vi "Main FPGA 5-axis with Limits.vi"() -> ()   [LabVIEW 2013]
uses:
  <vilib>/Motion/MotorControl/_s/nism.interpretControlRegister.stateTransition.ctl
  <vilib>/Platform/TimedLoop/XDataNode/timing_clust.ctl
  <vilib>/Platform/TimedLoop/XDataNode/nitl_modes.ctl
  <vilib>/Platform/TimedLoop/XDataNode/wakeup.ctl
  <vilib>/Motion/MotorControl/_s/nism.digitalInputs.portA.ctl
  <vilib>/rvi/Emulation/niFpgaSctlEmulationGetInTimedLoop.vi
  <vilib>/rvi/Emulation/niFpgaEmulationReportErrorSimple.vi
  <vilib>/rvi/Emulation/niFpgaGetClockAttributes.vi
  <vilib>/rvi/Emulation/niFpgaCriticalErrorInLSC.vi
  Global FPGA.vi
  <vilib>/rvi/eio/common/nirviEmuTemplateMethod_errors.vi
  <vilib>/Motion/SoftMotion/Synchronization/nism.rioScan.generateSyncScan.vi
  <vilib>/rvi/Emulation/niFpgaProcessEmulError.vi
  <vilib>/Motion/MotorControl/_s/nism.interpretControlRegister.indexed.vi
  <vilib>/Motion/MotorControl/_s/nism.generateStatusRegister.indexed.vi
  <vilib>/Motion/MotorControl/_s/nism.mdo.read.positionLoopSyncData.vi
  <vilib>/Motion/MotorControl/_s/nism.mdo.read.splineData.vi
  <vilib>/Motion/MotorControl/_s/nism.splineInterpolation.fxp.3.index.vi
  <vilib>/Motion/MotorControl/_s/nism.mdo.handler.indexed.vi
  <vilib>/Motion/MotorControl/_s/nism.digitalFilter.u8.vi
  <vilib>/Motion/MotorControl/_s/nism.interpretDIOControl.portA.single.2.vi
  <vilib>/Motion/MotorControl/_s/nism.generateDIOStatus.portA.single.vi
  <vilib>/Platform/TimedLoop/XDataNode/XDataNode.xnode
  <vilib>/eio/EIONode/EIONode.xnode
  <vilib>/Motion/MotorControl/NI_SoftMotion_MotorControlIP.lvlib
  <vilib>/Platform/TimedLoop/XDataNode/XDNodeRunTimeDep.lvlib
  <vilib>/Motion/SoftMotion/Synchronization/NI_SoftMotion_Synchronization.lvlib
panel:
  in  "Axis Digital Inputs (U8)":u8[](array[numeric])=[0, 0, 0, 0, 0, 0, 0, 0]
  out "Axis Positions":fxp<+/-,64,32>[](array[numeric])
  in  "STEP or CW? (T=STEP)":bool
  out "Drive Enable":bool[](array[boolean])
  in  "Enable Watchdog":bool
  in  "Pet Watchdog":bool
  in  "Watchdog Timeout Period (ticks)":u64=40000000 format="%.0p"
  out "Watchdog Timed Out?":bool
  out "Time Since Last Pet":u64
  in  "Enable value":bool
  in  "Drive Enable override?":bool
  out "State":T1=enum."Start --> Initializing" caption="state transition"
  in  "Sync Value":bool
  in  "Sync Enable override?":bool
  in  "Invert direction?":bool
  out "Sync is Fault":bool
  out "Sync is Locked":bool
  in  "minimum pulse":u16=40
  # "Synchronization Loop"
  # "Control Status Loop"
  # "Notes: \n1. This VI provides the communication interface between the NI SoftMotion Engine and the LabVIEW FPGA Module. You must compile this VI for a specific FPGA target before use. After compiling, run the VI before running any of the Express VI examples. For information on moving this example to another FPGA target, refer to ni.com/info and enter info code fpgaex.\n\n2. Only use the Reset Axis button if you are unable to communicate with the axis by any other means. This button resets the device state machine and other VIs to a known state. After resetting the axis, switch the NI Scan Engine from Active Mode to Configuration Mode, then back to Active Mode, before attempting to enable the axis."
  # "(These two buttons \nare for testing\npurposes.)"
  # "(These two buttons \nare for testing\npurposes.)"
  # "Step/Direction Loop"
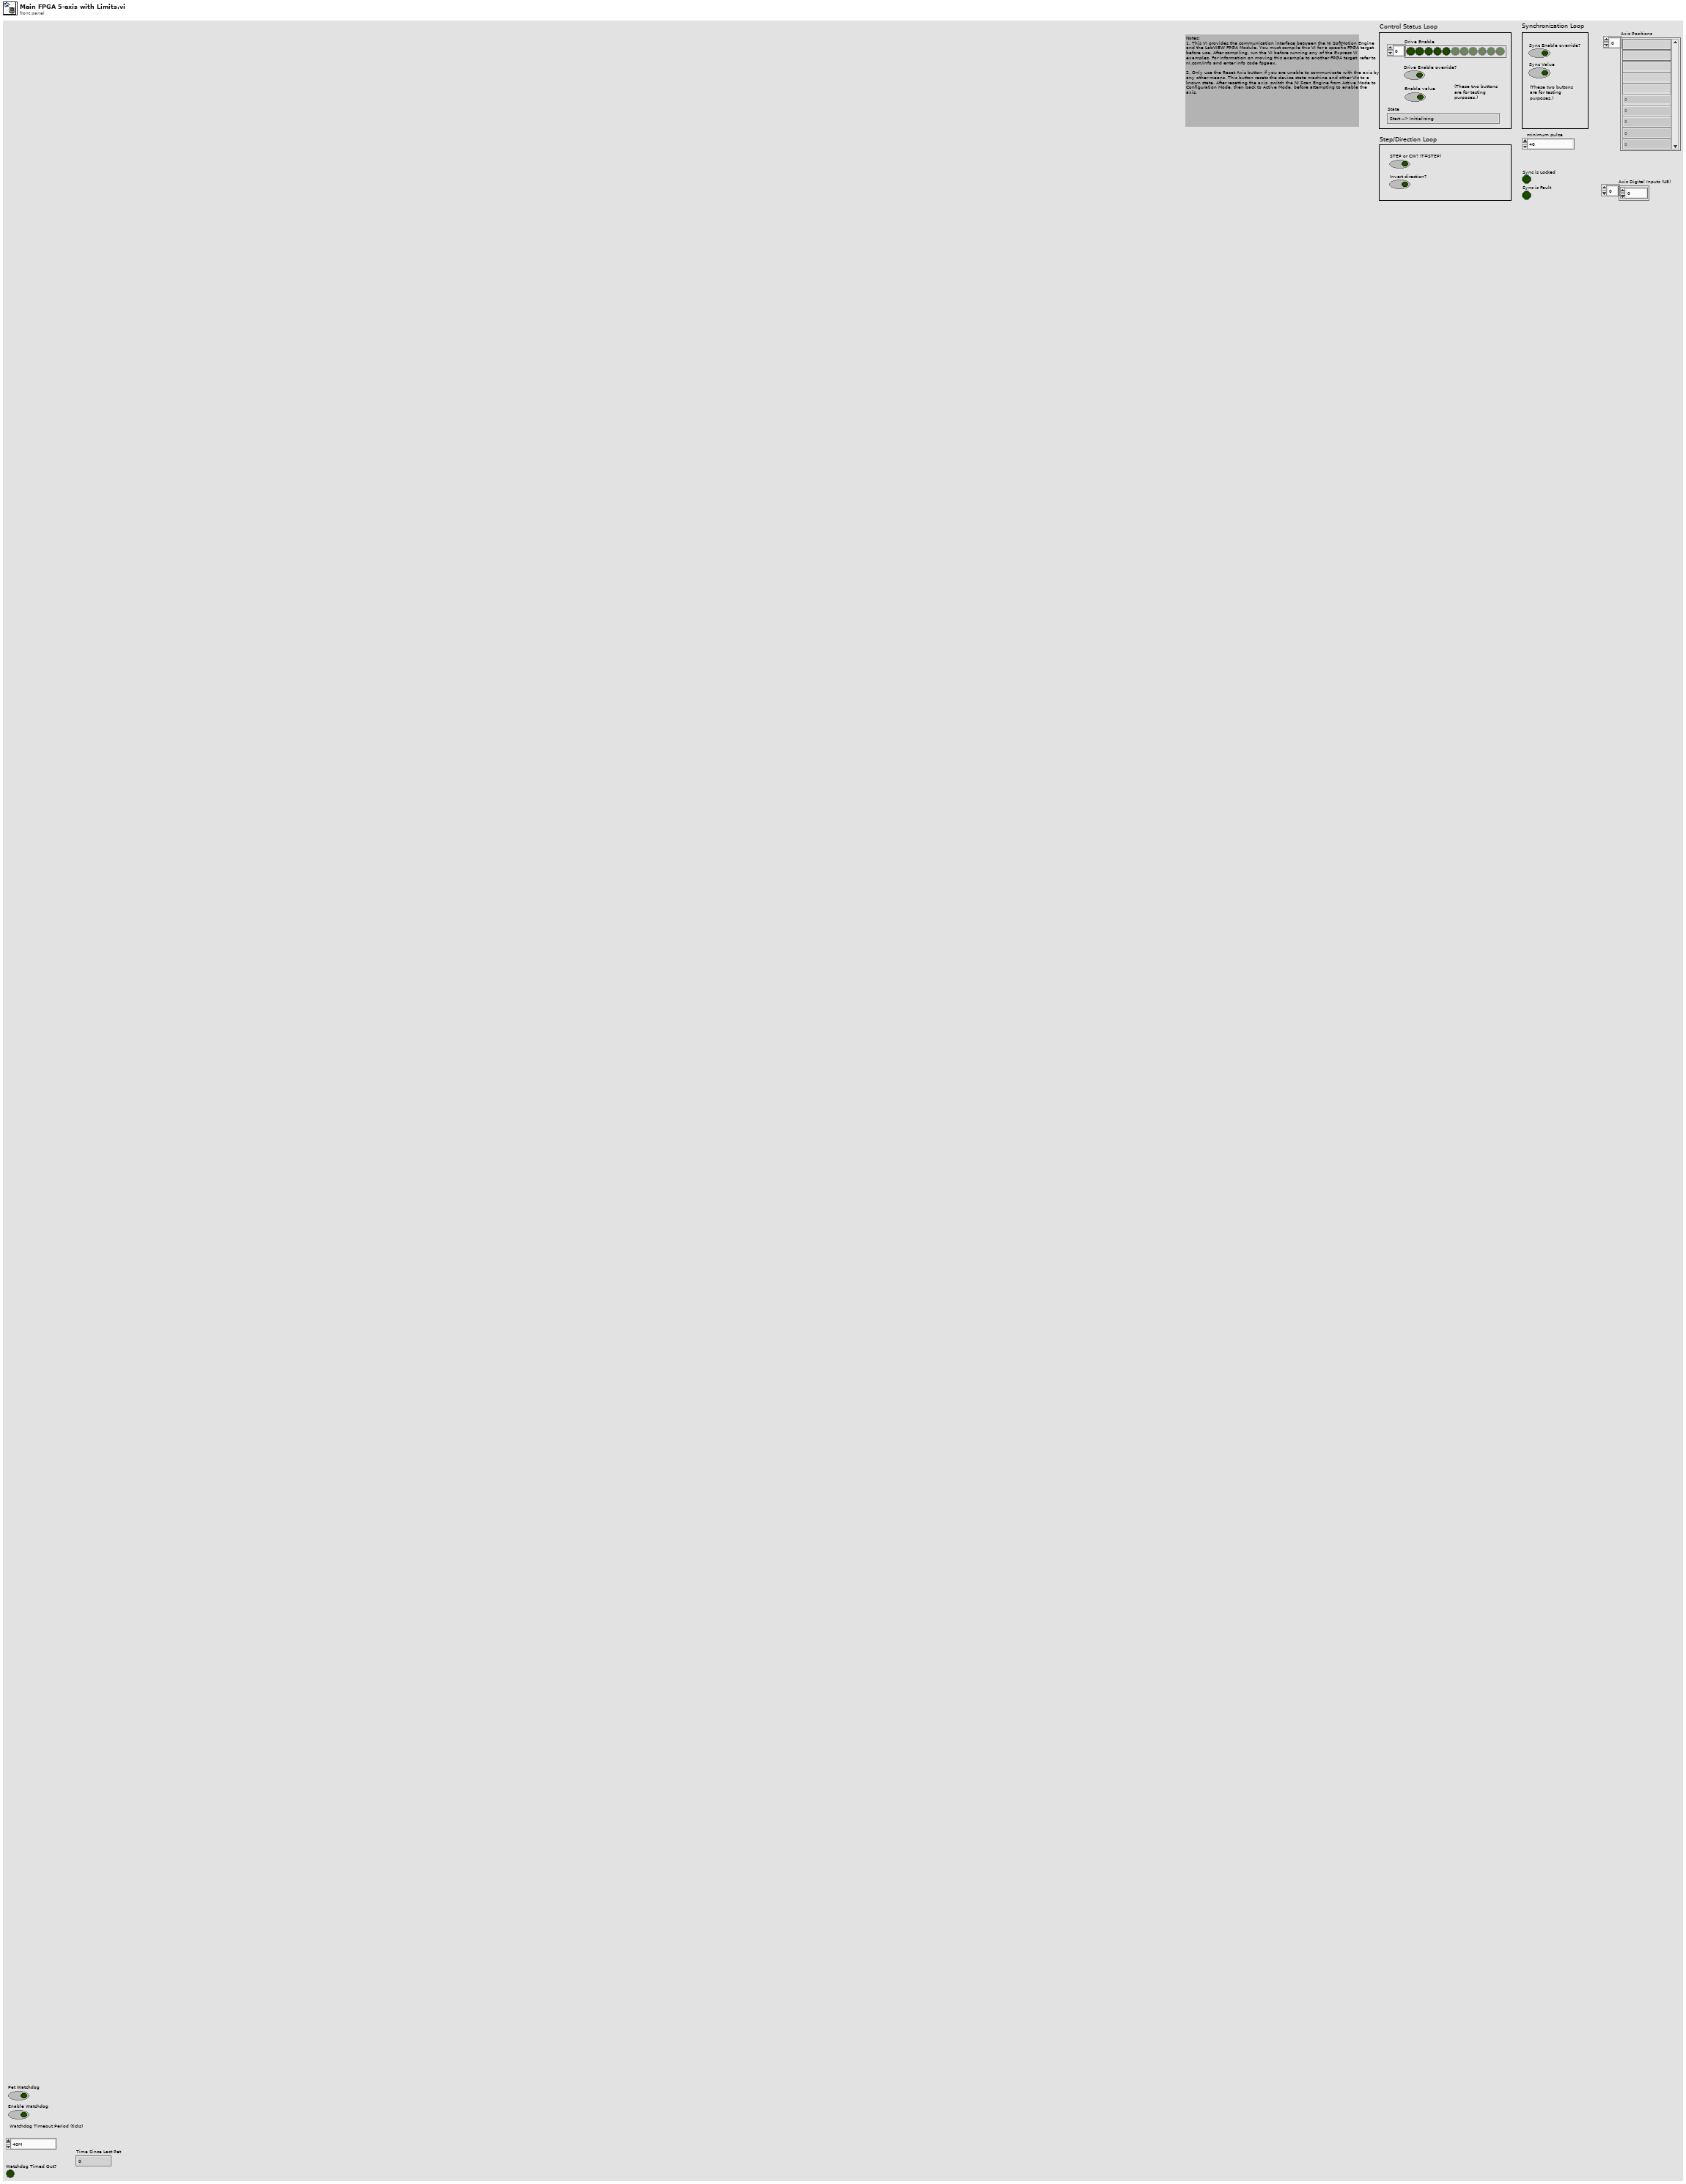
[diagram p1: front panel]
types:
  T1 = typedef "NI_SoftMotion_MotorControlIP.lvlib/nism.interpretControlRegister.stateTransition.ctl" = enum8{"Invalid", "Start --> Initializing", "Initializing --> Disabled", "Disabled --> Ready To Switch On", "Ready To Switch On --> Switched On", "Ready To Switch On --> Disable", "Switched On --> Operation Enable", "Switched On --> Ready To Switch On", "Switched On --> Disabled", "Operation Enable --> Switched On", "Operation Enable --> Ready To Switch On", "Operation Enable --> Disabled", "Fault --> Disabled", "Any --> Fault", "None"}
  T2 = typedef "NI_SoftMotion_MotorControlIP.lvlib/nism.mdo.splineData.ctl" = cluster{"spline type":T3, "traj per/spline per":u16, "spline per/traj per":fxp<+,32,0>}
  T3 = typedef "nism.splineInterpolation.type.ctl" = u16
  T4 = typedef "NI_SoftMotion_Synchronization.lvlib/nism.softmotionScan.timerConfig.ctl" = cluster{"Target Period (clocks)":u16, "Host Period / Target Period":u16}
  T5 = typedef "NI_SoftMotion_Synchronization.lvlib/nism.softmotionScan.timerControl.ctl" = cluster{"SM Scan":bool, "SM Scan Count":u32, "SM Scan Enabled":bool}
  T6 = typedef "XDNodeRunTimeDep.lvlib/timing_clust.ctl" = cluster{"Expected End [f-1]":u64, "Actual End [f-1]":u64, "Finished Late? [f-1]":bool, "Expected End [i-1]":u64, "Actual End [i-1]":u64, "Finished Late? [i-1]":bool, "Expected Start [i]":u64, "Actual Start [i]":u64, "Expected Start [f]":u64, "Actual Start [f]":u64, "Source Name":string, "Structure Name":string, "Period":i64, "Deadline":i64, "Offset":i64, "Start":i64, "Priority":i32, "Timeout":i32, "Mode":T7, "Wakeup Reason":T8, "Error":errorcluster, "Source Type":string, "Secondary Source Type":string, "Global End Time":u64, "Global Start Time":u64, "Frame Duration":u64, "Iteration Duration":u64, "Assigned CPU":i32, "I/O Scan Engine Mode":u32}
  T7 = typedef "XDNodeRunTimeDep.lvlib/nitl_modes.ctl" = enum32{"No Change", "Process missed periods, maintain original phase", "Discard missed periods, maintain original phase", "Process missed periods, ignore original phase", "Discard missed periods, ignore original phase"}
  T8 = typedef "XDNodeRunTimeDep.lvlib/wakeup.ctl" = enum32{"Normal", "Aborted", "Asynchronous wakeup", "Timing source error", "Timed loop error", "Timeout"}
  T9 = typedef "NI_SoftMotion_MotorControlIP.lvlib/nism.digitalInputs.portA.ctl" = cluster{"reverse limit":bool, "forward limit":bool, "home switch":bool, "digital input 0":bool, "digital input 1":bool, "digital input 2":bool, "digital input 3":bool}
  T10 = typedef "NI_SoftMotion_MotorControlIP.lvlib/nism.dio.portA.config.2.ctl" = cluster{"digital filter (us)":u16[], "safe state":enum16{"Low", "High", "No Change"}[]}
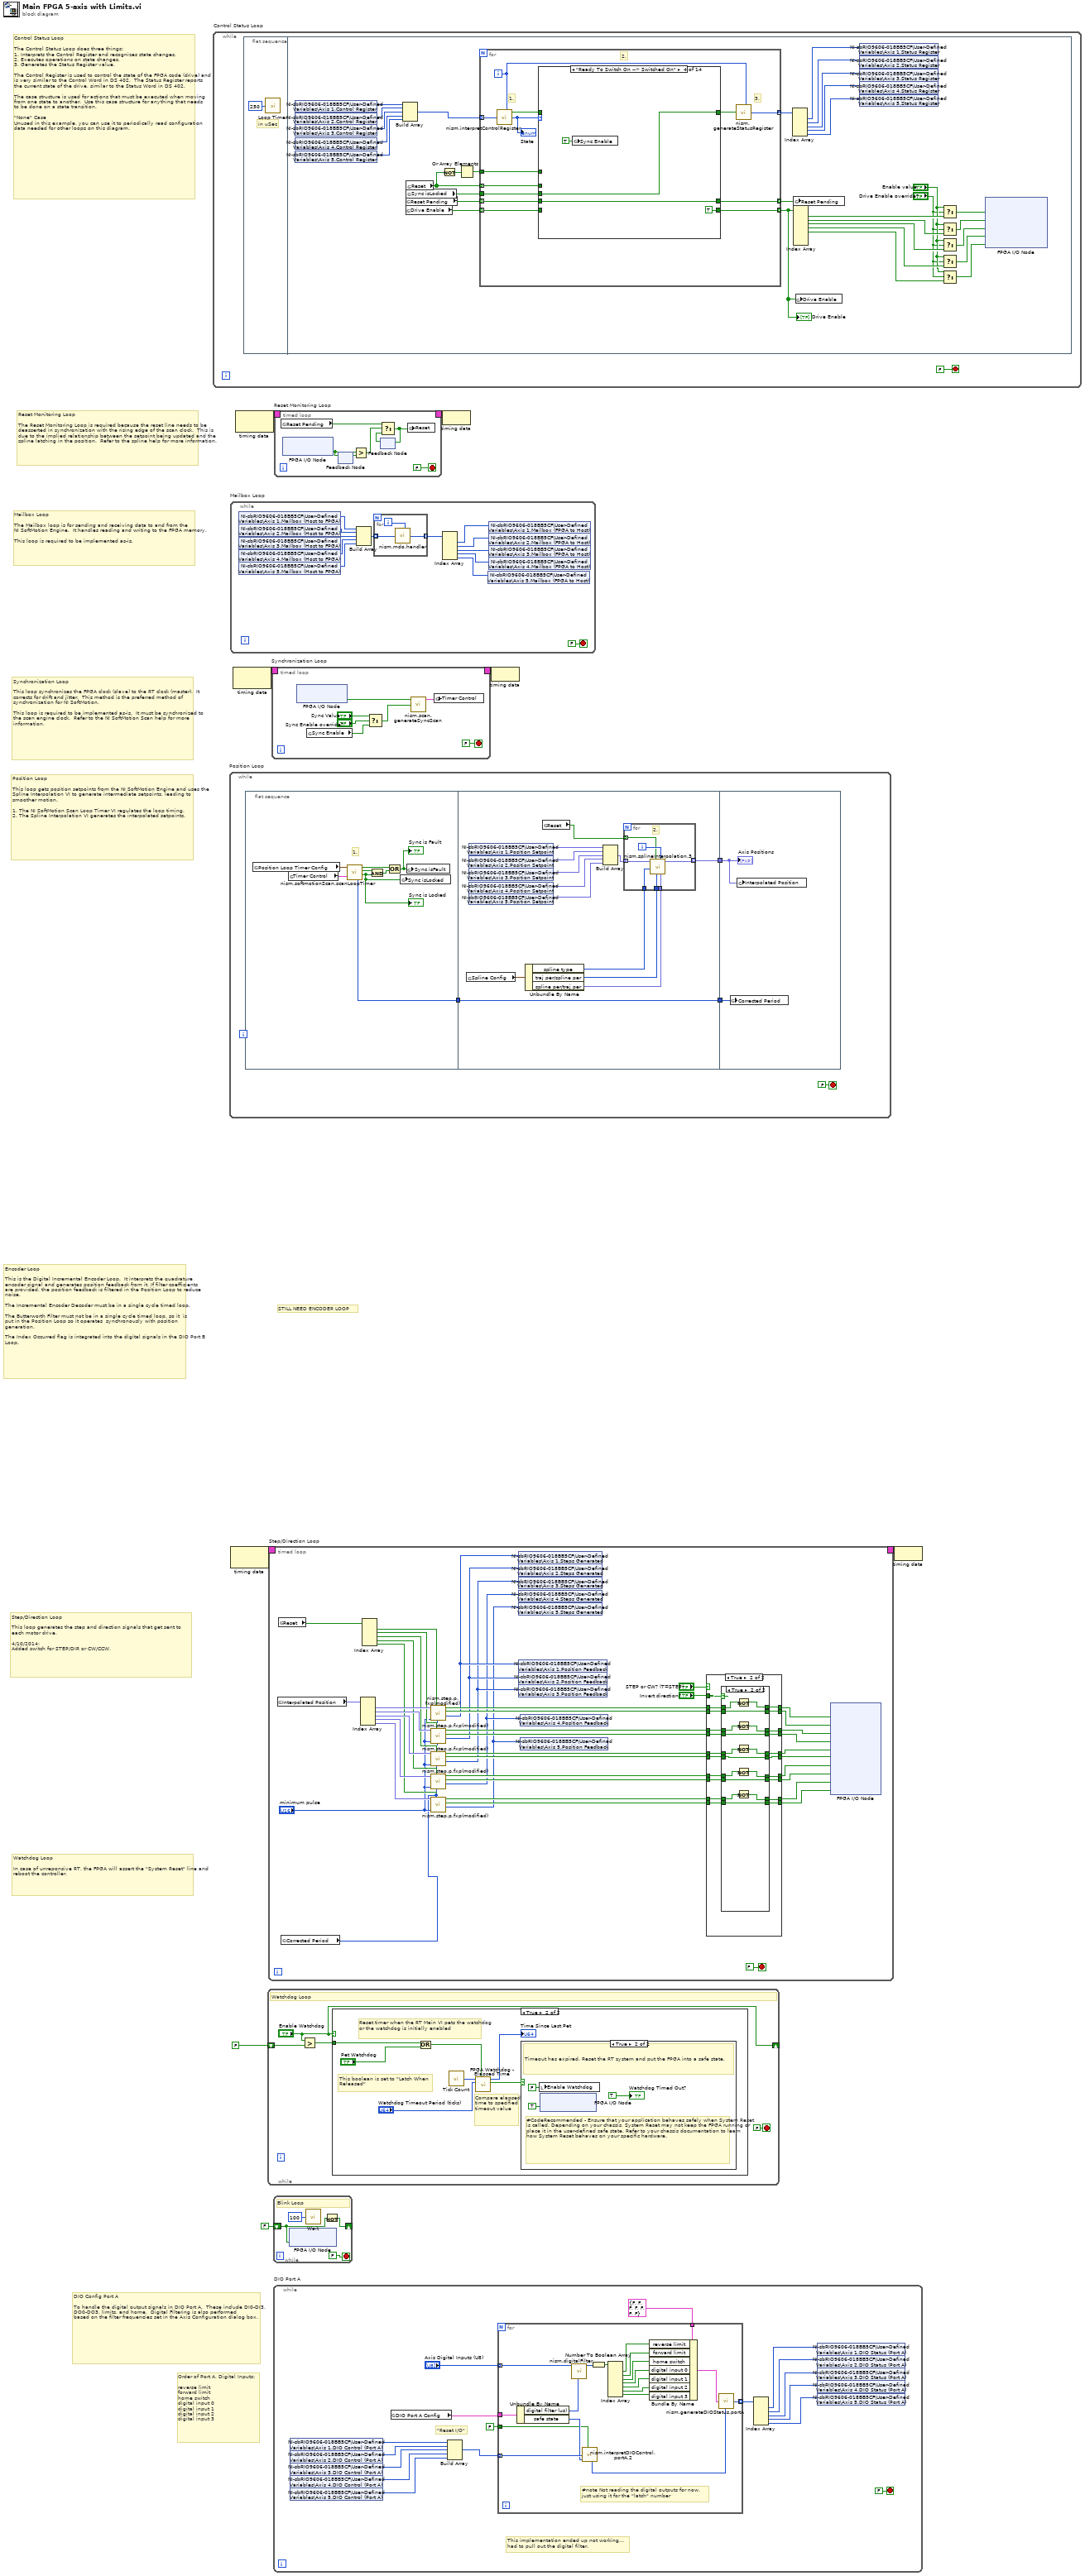
[diagram p0: block diagram]
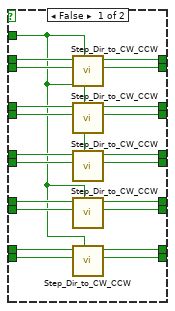
[diagram p4: hidden frame]
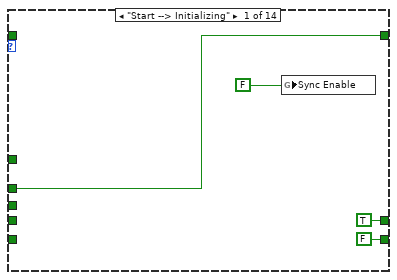
[diagram p6: hidden frame]
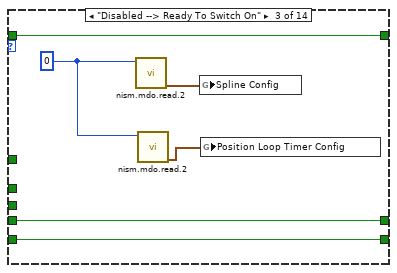
[diagram p8: hidden frame]
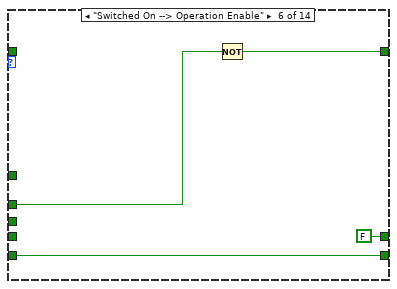
[diagram p10: hidden frame]
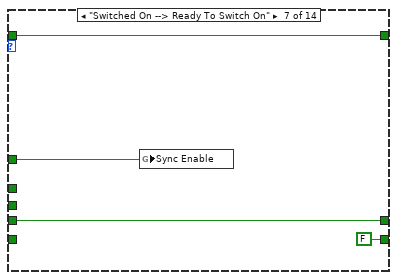
[diagram p11: hidden frame]
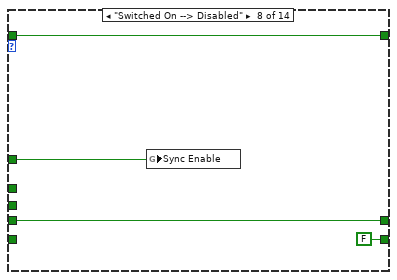
[diagram p12: hidden frame]
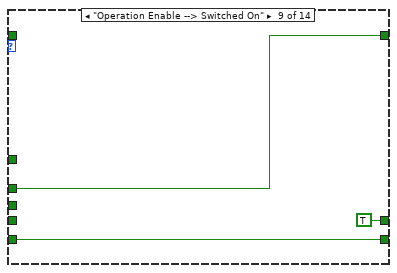
[diagram p13: hidden frame]
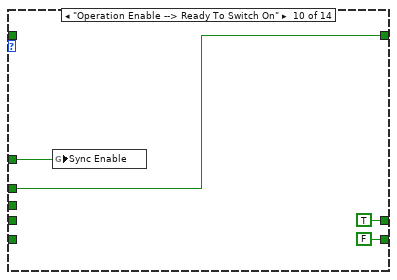
[diagram p14: hidden frame]
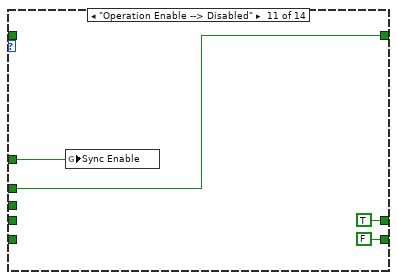
[diagram p15: hidden frame]
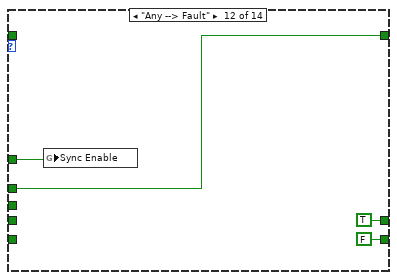
[diagram p16: hidden frame]
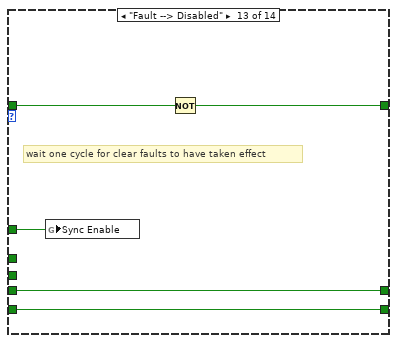
[diagram p17: hidden frame]
diagram:
  # "STILL NEED ENCODER LOOP"
  # "DIO Config Port A\n\nTo handle the digital output signals in DIO Port A.  These include DI0-DI3, DO0-DO3, limits, and home.  Digital Filtering is also performed\nbased on the filter frequencies set in the Axis Configuration dialog box."
  # "Order of Port A, Digital Inputs:\n\nreverse limit\nforward limit\nhome switch\ndigital input 0\ndigital input 1\ndigital input 2\ndigital input 3"
  # "Encoder Loop\n\nThis is the Digital Incremental Encoder Loop.  It interprets the quadrature encoder signal and generates position feedback from it. If filter coefficients are provided, the position feedback is filtered in the Position Loop to reduce noise.\n\nThe Incremental Encoder Decoder must be in a single cycle timed loop.\n\nThe Butterworth Filter must not be in a single cycle timed loop, so it  is\nput in the Position Loop so it operates  synchronously with position generation.\n\nThe Index Occurred flag is integrated into the digital signals in the DIO Port B Loop."
  # "Watchdog Loop\n\nIn case of unreponsive RT, the FPGA will assert the \"System Reset\" line and reboot the controller."
  # "Step/Direction Loop\n\nThis loop generates the step and direction signals that get sent to \neach motor drive.\n\n4/10/2014:\nAdded switch for STEP/DIR or CW/CCW."
  # "Position Loop\n\nThis loop gets position setpoints from the NI SoftMotion Engine and uses the Spline Interpolation VI to generate intermediate setpoints, leading to smoother motion.\n\n1. The NI SoftMotion Scan Loop Timer VI regulates the loop timing. \n2. The Spline Interpolation VI generates the interpolated setpoints."
  # "Synchronization Loop\n\nThis loop synchronizes the FPGA clock (slave) to the RT clock (master).  It corrects for drift and jitter.  This method is the preferred method of synchronization for NI SoftMotion.\n\nThis loop is required to be implemented as-is.  It must be synchronized to the scan engine clock.  Refer to the NI SoftMotion Scan help for more information."
  # "Mailbox Loop\n\nThe Mailbox loop is for sending and receiving data to and from the \nNI SoftMotion Engine.  It handles reading and writing to the FPGA memory.\n\nThis loop is required to be implemented as-is."
  # "Reset Monitoring Loop\n\nThe Reset Monitoring Loop is required because the reset line needs to be deasserted in synchronization with the rising edge of the scan clock.  This is due to the implied relationship between the setpoint being updated and the spline latching in the position.  Refer to the spline help for more information."
  # "Control Status Loop\n\nThe Control Status Loop does three things:\n1. Interprets the Control Register and recognizes state changes.\n2. Executes operations on state changes.\n3. Generates the Status Register value.\n\nThe Control Register is used to control the state of the FPGA code (drive) and is very similar to the Control Word in DS 402.  The Status Register reports the current state of the drive, similar to the Status Word in DS 402.\n\nThe case structure is used for actions that must be executed when moving from one state to another.  Use this case structure for anything that needs to be done on a state transition.\n\n\"None\" Case\nUnused in this example, you can use it to periodically read configuration data needed for other loops on this diagram."
  n1 = while "Control Status Loop" {
    stop <- FALSE stop-if-true
    n2 = flat-sequence {
      frame #0 {
        # "in uSec"
        n3 = call "Loop Timer"("Count(uSec)"=u32 250) -> ()  [unwired: 1 out]
      }
      frame #1 {
        n4 = shared-variable "NI-sbRIO9606-018BB5CF\\User-Defined Variables\\Axis 1.Control Register"() -> (w32:u32)  [unwired: 1 in, 1 out]
        n5 = shared-variable "NI-sbRIO9606-018BB5CF\\User-Defined Variables\\Axis 2.Control Register"() -> (w31:u32)  [unwired: 1 in, 1 out]
        n6 = shared-variable "NI-sbRIO9606-018BB5CF\\User-Defined Variables\\Axis 3.Control Register"() -> (w30:u32)  [unwired: 1 in, 1 out]
        n7 = shared-variable "NI-sbRIO9606-018BB5CF\\User-Defined Variables\\Axis 4.Control Register"() -> (w29:u32)  [unwired: 1 in, 1 out]
        n8 = shared-variable "NI-sbRIO9606-018BB5CF\\User-Defined Variables\\Axis 5.Control Register"() -> (w28:u32)  [unwired: 1 in, 1 out]
        n9 = Build Array(w32, w31, w30, w29, w28) -> (w41:u32[])
        n10 = global read "Global FPGA.vi" "Reset Pending"() -> (w36:bool[])
        n11 = global read "Global FPGA.vi" "Drive Enable"() -> (w35:bool[])
        n12 = global read "Global FPGA.vi" "Reset"() -> (w37:bool[])
        n13 = global read "Global FPGA.vi" "Sync isLocked"() -> (w42:bool)
        n14 = Not(x=w37) -> (.not. x?=w39:bool[])
        n15 = Or Array Elements(Boolean array=w39) -> (logical OR=w38:bool)
        n16 = for {
          tunnel: w37 -> [w50] mode=indexing
          tunnel: w42 -> [w49]
          tunnel: w41 -> [w51] mode=indexing
          tunnel: [w48] -> w33 mode=indexing
          tunnel: [w47] -> w40 mode=indexing
          tunnel: [w46] -> w34 mode=indexing
          tunnel: w38 -> [w45]
          tunnel: w36 -> [w44] mode=indexing
          tunnel: w35 -> [w43] mode=indexing
          i -> [w52]
          # "3."
          # "2."
          # "1."
          n17 = call-poly <vilib>:"nism.interpretControlRegister.vi"("control register"=w51, "axis index"=w52) -> ("transition occurred"=w53:bool, "state transition"=w54:T1)  [unwired: 6 in]
          "State" <- w54
          n18 = case shown="\"Ready To Switch On --> Switched On\"" w54 {
            tunnel: w53 -> [_ w62 w68 _ w75 _ w83 w87 _ _ _ _ w107 _]
            tunnel: [w59 w62 w68 w70 w75 w79 w83 w87 w89 w92 w96 w100 w106 _] -> w55
            tunnel: w50 -> [w59 _ _ _ _ w78 _ _ w89 w92 w96 w100 _ _]
            tunnel: w49 -> [_ _ _ w70 _ _ _ _ _ _ _ _ _ _]
            tunnel: [TRUE ("Write.Reset Pending") w61 w64 w69 w74 FALSE ("Write.Reset Pending") w80 w84 TRUE ("Write.Reset Pending") TRUE ("Write.Reset Pending") TRUE ("Write.Reset Pending") TRUE ("Write.Reset Pending") w104 w109] -> w47
            tunnel: [FALSE ("Write.Drive Enable") w60 w63 TRUE ("Write.Drive Enable") w73 w76 FALSE ("Write.Drive Enable") FALSE ("Write.Drive Enable") w88 FALSE ("Write.Drive Enable") FALSE ("Write.Drive Enable") FALSE ("Write.Drive Enable") w103 w108] -> w46
            tunnel: w45 -> [_ _ _ _ _ _ w81 w85 _ w91 w95 w99 w105 _]
            tunnel: w44 -> [_ w61 w64 w69 w74 _ w80 w84 _ _ _ _ w104 w109]
            tunnel: w43 -> [_ w60 w63 _ w73 w76 _ _ w88 _ _ _ w103 w108]
            frame "Start --> Initializing" {
              n19 = global write "Global FPGA.vi" "Sync Enable"(FALSE ("Sync Enable")) -> ()
            }
            frame "Initializing --> Disabled" {
            }
            frame "Disabled --> Ready To Switch On" {
              w66 = 0 ("axis index")
              n20 = call-poly <vilib>:"nism.mdo.read.2.vi"("axis index"=w66) -> ("spline"=w67:T2)  [unwired: 10 in]
              n21 = call-poly <vilib>:"nism.mdo.read.2.vi"("axis index"=w66) -> ("position loop sync"=w65:T4)  [unwired: 10 in]
              n22 = global write "Global FPGA.vi" "Spline Config"(w67) -> ()
              n23 = global write "Global FPGA.vi" "Position Loop Timer Config"(w65) -> ()
            }
            frame "Ready To Switch On --> Switched On" {
              n24 = global write "Global FPGA.vi" "Sync Enable"(TRUE ("Sync Enable")) -> ()
            }
            frame "Ready To Switch On --> Disable" {
            }
            frame "Switched On --> Operation Enable" {
              n25 = Not(x=w78) -> (.not. x?=w79:bool)
            }
            frame "Switched On --> Ready To Switch On" {
              n26 = global write "Global FPGA.vi" "Sync Enable"(w81) -> ()
            }
            frame "Switched On --> Disabled" {
              n27 = global write "Global FPGA.vi" "Sync Enable"(w85) -> ()
            }
            frame "Operation Enable --> Switched On" {
            }
            frame "Operation Enable --> Ready To Switch On" {
              n28 = global write "Global FPGA.vi" "Sync Enable"(w91) -> ()
            }
            frame "Operation Enable --> Disabled" {
              n29 = global write "Global FPGA.vi" "Sync Enable"(w95) -> ()
            }
            frame "Any --> Fault" {
              n30 = global write "Global FPGA.vi" "Sync Enable"(w99) -> ()
            }
            frame "Fault --> Disabled" {
              # "wait one cycle for clear faults to have taken effect"
              n31 = global write "Global FPGA.vi" "Sync Enable"(w105) -> ()
              n32 = Not(x=w107) -> (.not. x?=w106:bool)
            }
            frame "None", Default {
            }
          }
          n33 = call-poly <vilib>:"nism.generateStatusRegister.vi"("transition success"=w55, "axis index"=w52) -> ("status register"=w48:u32)  [unwired: 7 in]
        }
        "Drive Enable" <- w34
        n34 = Index Array(array=w33) -> (element #1=w27:u32, element #2=w26:u32, element #3=w25:u32, element #4=w24:u32, element #5=w23:u32)  [unwired: 5 in]
        n35 = global write "Global FPGA.vi" "Reset Pending"(w40) -> ()
        n36 = Index Array(array=w34) -> (element #1=w22:bool, element #2=w20:bool, element #3=w18:bool, element #4=w16:bool, element #5=w14:bool)  [unwired: 8 in, 3 out]
        n37 = global write "Global FPGA.vi" "Drive Enable"(w34) -> ()
        n38 = shared-variable "NI-sbRIO9606-018BB5CF\\User-Defined Variables\\Axis 1.Status Register"(w27) -> ()  [unwired: 1 in, 1 out]
        n39 = shared-variable "NI-sbRIO9606-018BB5CF\\User-Defined Variables\\Axis 2.Status Register"(w26) -> ()  [unwired: 1 in, 1 out]
        n40 = shared-variable "NI-sbRIO9606-018BB5CF\\User-Defined Variables\\Axis 3.Status Register"(w25) -> ()  [unwired: 1 in, 1 out]
        n41 = shared-variable "NI-sbRIO9606-018BB5CF\\User-Defined Variables\\Axis 4.Status Register"(w24) -> ()  [unwired: 1 in, 1 out]
        n42 = shared-variable "NI-sbRIO9606-018BB5CF\\User-Defined Variables\\Axis 5.Status Register"(w23) -> ()  [unwired: 1 in, 1 out]
        n43 = Select(t="Enable value", s="Drive Enable override?", f=w22) -> (s? t:f=w21:bool)
        n44 = Select(t="Enable value", s="Drive Enable override?", f=w20) -> (s? t:f=w19:bool)
        n45 = Select(t="Enable value", s="Drive Enable override?", f=w18) -> (s? t:f=w17:bool)
        n46 = Select(t="Enable value", s="Drive Enable override?", f=w16) -> (s? t:f=w15:bool)
        n47 = Select(t="Enable value", s="Drive Enable override?", f=w14) -> (s? t:f=w13:bool)
        n48 = xnode "FPGA I/O Node"("Axis1_Servo On"=w21, "Axis2_Servo On"=w19, "Axis3_Servo On"=w17, "Axis4_Servo On"=w15, "Axis5_Servo On"=w13) -> ()  [unwired: 5 in, 5 out]
      }
    }
  }
  n49 = while "Position Loop" {
    stop <- FALSE stop-if-true
    n50 = flat-sequence {
      tunnel: [w114] -> w110
      tunnel: [w128] -> w112
      tunnel: [w127] -> w111
      tunnel: w110 -> [w127]
      tunnel: w112 -> [w142]
      tunnel: w111 -> [w143]
      frame #0 {
        # "1."
        n51 = global read "Global FPGA.vi" "Position Loop Timer Config"() -> (w116:T4)
        n52 = global read "Global FPGA.vi" "Timer Control"() -> (w115:T5)
        n53 = call <vilib>:"nism.softmotionScan.scanLoopTimer.vi"("Timer Control"=w115, "Timer Config"=w116) -> ("Scan Running?"=w118:bool, "Finished Late?"=w120:bool, "Fault Occurred?"=w121:bool, "Corrected Period"=w114:u16)  [unwired: 5 in, 1 out]
        "Sync is Locked" <- w118
        n54 = Compound Arithmetic op=AND(w120, w118) -> (w119:bool)
        n55 = Compound Arithmetic op=OR(w121, w119) -> (w117:bool)
        "Sync is Fault" <- w117
        n56 = global write "Global FPGA.vi" "Sync isLocked"(w118) -> ()
        n57 = global write "Global FPGA.vi" "Sync isFault"(w117) -> ()
      }
      frame #1 {
        n58 = global read "Global FPGA.vi" "Spline Config"() -> (w130:T2)
        n59 = shared-variable "NI-sbRIO9606-018BB5CF\\User-Defined Variables\\Axis 1.Position Setpoint"() -> (w126:fxp<+/-,64,32>)  [unwired: 1 in, 1 out]
        n60 = shared-variable "NI-sbRIO9606-018BB5CF\\User-Defined Variables\\Axis 2.Position Setpoint"() -> (w125:fxp<+/-,64,32>)  [unwired: 1 in, 1 out]
        n61 = shared-variable "NI-sbRIO9606-018BB5CF\\User-Defined Variables\\Axis 3.Position Setpoint"() -> (w124:fxp<+/-,64,32>)  [unwired: 1 in, 1 out]
        n62 = shared-variable "NI-sbRIO9606-018BB5CF\\User-Defined Variables\\Axis 4.Position Setpoint"() -> (w123:fxp<+/-,64,32>)  [unwired: 1 in, 1 out]
        n63 = shared-variable "NI-sbRIO9606-018BB5CF\\User-Defined Variables\\Axis 5.Position Setpoint"() -> (w122:fxp<+/-,64,32>)  [unwired: 1 in, 1 out]
        n64 = Unbundle By Name(w130) -> ("spline type"=w134:T3, "traj per/spline per"=w133:u16, "spline per/traj per"=w132:fxp<+,32,0>)
        n65 = global read "Global FPGA.vi" "Reset"() -> (w129:bool[])
        n66 = Build Array(w126, w125, w124, w123, w122) -> (w131:fxp<+/-,64,32>[])
        n67 = for {
          tunnel: w134 -> [w141]
          tunnel: w133 -> [w140]
          tunnel: w132 -> [w139]
          tunnel: w129 -> [w136] mode=indexing
          tunnel: w131 -> [w138] mode=indexing
          tunnel: [w135] -> w128 mode=indexing
          i -> [w137]
          # "2."
          n68 = call-poly <vilib>:"nism.splineInterpolation.3.vi"("1 / calls per sample"=w139, "index"=w137, "calls per sample"=w140, "reset"=w136, "spline type"=w141, "x"=w138) -> ("xi"=w135:fxp<+/-,64,32>)  [unwired: 5 in]
        }
      }
      frame #2 {
        n69 = global write "Global FPGA.vi" "Corrected Period"(w143) -> ()
        n70 = global write "Global FPGA.vi" "Interpolated Position"(w142) -> ()
        "Axis Positions" <- w142
      }
    }
  }
  n71 = while "Mailbox Loop" {
    stop <- FALSE stop-if-true
    n72 = shared-variable "NI-sbRIO9606-018BB5CF\\User-Defined Variables\\Axis 1.Mailbox (Host to FPGA)"() -> (w153:u64)  [unwired: 1 in, 1 out]
    n73 = shared-variable "NI-sbRIO9606-018BB5CF\\User-Defined Variables\\Axis 2.Mailbox (Host to FPGA)"() -> (w152:u64)  [unwired: 1 in, 1 out]
    n74 = shared-variable "NI-sbRIO9606-018BB5CF\\User-Defined Variables\\Axis 3.Mailbox (Host to FPGA)"() -> (w151:u64)  [unwired: 1 in, 1 out]
    n75 = shared-variable "NI-sbRIO9606-018BB5CF\\User-Defined Variables\\Axis 4.Mailbox (Host to FPGA)"() -> (w150:u64)  [unwired: 1 in, 1 out]
    n76 = shared-variable "NI-sbRIO9606-018BB5CF\\User-Defined Variables\\Axis 5.Mailbox (Host to FPGA)"() -> (w149:u64)  [unwired: 1 in, 1 out]
    n77 = Build Array(w153, w152, w151, w150, w149) -> (w155:u64[])
    n78 = for {
      tunnel: w155 -> [w159] mode=indexing
      tunnel: [w158] -> w154 mode=indexing
      i -> [w157]
      n79 = call-poly <vilib>:"nism.mdo.handler.vi"("mbox (host to fpga)"=w159, "axis index"=w157) -> ("mbox (fpga to host)"=w158:u64)  [unwired: 7 in]
    }
    n80 = Index Array(array=w154) -> (element #1=w148:u64, element #2=w147:u64, element #3=w146:u64, element #4=w145:u64, element #5=w144:u64)  [unwired: 5 in]
    n81 = shared-variable "NI-sbRIO9606-018BB5CF\\User-Defined Variables\\Axis 5.Mailbox (FPGA to Host)"(w144) -> ()  [unwired: 1 in, 1 out]
    n82 = shared-variable "NI-sbRIO9606-018BB5CF\\User-Defined Variables\\Axis 1.Mailbox (FPGA to Host)"(w148) -> ()  [unwired: 1 in, 1 out]
    n83 = shared-variable "NI-sbRIO9606-018BB5CF\\User-Defined Variables\\Axis 2.Mailbox (FPGA to Host)"(w147) -> ()  [unwired: 1 in, 1 out]
    n84 = shared-variable "NI-sbRIO9606-018BB5CF\\User-Defined Variables\\Axis 3.Mailbox (FPGA to Host)"(w146) -> ()  [unwired: 1 in, 1 out]
    n85 = shared-variable "NI-sbRIO9606-018BB5CF\\User-Defined Variables\\Axis 4.Mailbox (FPGA to Host)"(w145) -> ()  [unwired: 1 in, 1 out]
  }
  n86 = node-c288() -> (w8:T6)  [unwired: 1 in]
  n87 = node-c288() -> (w6:T6)  [unwired: 1 in]
  n88 = node-c288() -> (w4:T6)  [unwired: 1 in]
  n89 = while "RT Watchdog Loop" {
    shift-right: ["Enable Watchdog"] -> _
    shift-left: FALSE ("Enable RT Watchdog") -> [w163]
    stop <- FALSE stop-if-true
    # "Watchdog Loop"
    n90 = Greater?(x="Enable Watchdog", y=w163) -> (0:w160:bool)
    n91 = case shown="True" "Enable Watchdog" {
      tunnel: w160 -> [_ w166]
      frame False {
        # "This loop has to be explicitly enabled from the RT Main VI.  This reduces the possiblity of an endless reboot cycle."
      }
      frame True {
        # "This boolean is set to \"Latch When Released\""
        # "Compare elapsed time to specified timeout value"
        # "Reset timer when the RT Main VI pets the watchdog or the watchdog is initially enabled"
        n92 = Or(x=w166, y="Pet Watchdog") -> (x .or. y?=w165:bool)
        n93 = call "Tick Count"() -> ("Tick Count(Ticks)"=w169:u32)
        n94 = call "FPGA Watchdog - Elapsed Time.vi"("Reset"=w165, "Timeout Period"="Watchdog Timeout Period (ticks)", "Current Time"=w169) -> ("Timeout"=w164:bool, "Elapsed Time"=→"Time Since Last Pet":u64)  [unwired: 7 in]
        n95 = case shown="True" w164 {
          frame False {
            # "Timeout has not expired."
          }
          frame True {
            # "#CodeRecommended - Ensure that your application behaves safely when System Reset is called. Depending on your chassis, System Reset may not keep the FPGA running or place it in the user-defined safe state. Refer to your chassis documentation to learn how System Reset behaves on your specific hardware."
            # "Timeout has expired. Reset the RT system and put the FPGA into a safe state."
            n96 = local write "Enable Watchdog"(FALSE ("Enable RT Watchdog")) -> ()
            n97 = xnode "FPGA I/O Node"("System Reset"=TRUE ("RT Reset on Watchdog Failure?")) -> ()  [unwired: 1 in, 1 out]
            "Watchdog Timed Out?" <- TRUE ("Watchdog Timed Out?")
          }
        }
      }
    }
  }
  n98 = timed-loop "Step/Direction Loop" {
    timing: w8 -> [_]
    timing-out: [_] -> w7
    stop <- FALSE stop-if-true
    n99 = global read "Global FPGA.vi" "Interpolated Position"() -> (w214:fxp<+/-,64,32>[])
    n100 = global read "Global FPGA.vi" "Reset"() -> (w208:bool[])
    n101 = global read "Global FPGA.vi" "Corrected Period"() -> (w174:u16)
    n102 = Index Array(array=w214) -> (element #1=w213:fxp<+/-,64,32>, element #2=w212:fxp<+/-,64,32>, element #3=w211:fxp<+/-,64,32>, element #4=w210:fxp<+/-,64,32>, element #5=w209:fxp<+/-,64,32>)  [unwired: 5 in]
    n103 = Index Array(array=w208) -> (element #1=w207:bool, element #2=w206:bool, element #3=w205:bool, element #4=w204:bool, element #5=w203:bool)  [unwired: 5 in]
    n104 = call "nism.step.p.fxp(modified).vi"("calls per sample"=w174, "reset"=w207, "minimum pulse"="minimum pulse", "position setpoint"=w213) -> ("steps generated"=w179:i32, "step"=w201:bool, "direction"=w202:bool)  [unwired: 4 in, 1 out]
    n105 = call "nism.step.p.fxp(modified).vi"("calls per sample"=w174, "reset"=w206, "minimum pulse"="minimum pulse", "position setpoint"=w212) -> ("steps generated"=w178:i32, "step"=w199:bool, "direction"=w200:bool)  [unwired: 4 in, 1 out]
    n106 = call "nism.step.p.fxp(modified).vi"("calls per sample"=w174, "reset"=w205, "minimum pulse"="minimum pulse", "position setpoint"=w211) -> ("steps generated"=w177:i32, "step"=w197:bool, "direction"=w198:bool)  [unwired: 4 in, 1 out]
    n107 = call "nism.step.p.fxp(modified).vi"("calls per sample"=w174, "reset"=w204, "minimum pulse"="minimum pulse", "position setpoint"=w210) -> ("steps generated"=w176:i32, "step"=w195:bool, "direction"=w196:bool)  [unwired: 4 in, 1 out]
    n108 = call "nism.step.p.fxp(modified).vi"("calls per sample"=w174, "reset"=w203, "minimum pulse"="minimum pulse", "position setpoint"=w209) -> ("steps generated"=w175:i32, "step"=w193:bool, "direction"=w194:bool)  [unwired: 4 in, 1 out]
    n109 = shared-variable "NI-sbRIO9606-018BB5CF\\User-Defined Variables\\Axis 1.Steps Generated"(w179) -> ()  [unwired: 1 in, 1 out]
    n110 = shared-variable "NI-sbRIO9606-018BB5CF\\User-Defined Variables\\Axis 2.Steps Generated"(w178) -> ()  [unwired: 1 in, 1 out]
    n111 = shared-variable "NI-sbRIO9606-018BB5CF\\User-Defined Variables\\Axis 3.Steps Generated"(w177) -> ()  [unwired: 1 in, 1 out]
    n112 = shared-variable "NI-sbRIO9606-018BB5CF\\User-Defined Variables\\Axis 4.Steps Generated"(w176) -> ()  [unwired: 1 in, 1 out]
    n113 = shared-variable "NI-sbRIO9606-018BB5CF\\User-Defined Variables\\Axis 5.Steps Generated"(w175) -> ()  [unwired: 1 in, 1 out]
    n114 = shared-variable "NI-sbRIO9606-018BB5CF\\User-Defined Variables\\Axis 1.Position Feedback"(w179) -> ()  [unwired: 1 in, 1 out]
    n115 = shared-variable "NI-sbRIO9606-018BB5CF\\User-Defined Variables\\Axis 2.Position Feedback"(w178) -> ()  [unwired: 1 in, 1 out]
    n116 = shared-variable "NI-sbRIO9606-018BB5CF\\User-Defined Variables\\Axis 3.Position Feedback"(w177) -> ()  [unwired: 1 in, 1 out]
    n117 = shared-variable "NI-sbRIO9606-018BB5CF\\User-Defined Variables\\Axis 4.Position Feedback"(w176) -> ()  [unwired: 1 in, 1 out]
    n118 = shared-variable "NI-sbRIO9606-018BB5CF\\User-Defined Variables\\Axis 5.Position Feedback"(w175) -> ()  [unwired: 1 in, 1 out]
    n119 = case shown="True" "STEP or CW? (T=STEP)" {
      tunnel: w202 -> [w236 w256]
      tunnel: w201 -> [w235 w246]
      tunnel: w200 -> [w234 w254]
      tunnel: w199 -> [w233 w244]
      tunnel: w198 -> [w232 w252]
      tunnel: w197 -> [w231 w242]
      tunnel: w196 -> [w230 w250]
      tunnel: w195 -> [w229 w240]
      tunnel: w194 -> [w228 w248]
      tunnel: w193 -> [w227 w238]
      tunnel: "Invert direction?" -> [w216 w257]
      tunnel: [w226 w255] -> w191
      tunnel: [w225 w245] -> w182
      tunnel: [w224 w253] -> w190
      tunnel: [w223 w243] -> w189
      tunnel: [w222 w251] -> w188
      tunnel: [w221 w241] -> w187
      tunnel: [w220 w249] -> w186
      tunnel: [w219 w239] -> w185
      tunnel: [w218 w247] -> w184
      tunnel: [w217 w237] -> w183
      frame False {
        n120 = call "Step_Dir_to_CW_CCW.vi"("invert"=w216, "step"=w235, "direction"=w236) -> ("CCW"=w225:bool, "CW"=w226:bool)  [unwired: 7 in]
        n121 = call "Step_Dir_to_CW_CCW.vi"("invert"=w216, "step"=w233, "direction"=w234) -> ("CCW"=w223:bool, "CW"=w224:bool)  [unwired: 7 in]
        n122 = call "Step_Dir_to_CW_CCW.vi"("invert"=w216, "step"=w231, "direction"=w232) -> ("CCW"=w221:bool, "CW"=w222:bool)  [unwired: 7 in]
        n123 = call "Step_Dir_to_CW_CCW.vi"("invert"=w216, "step"=w229, "direction"=w230) -> ("CCW"=w219:bool, "CW"=w220:bool)  [unwired: 7 in]
        n124 = call "Step_Dir_to_CW_CCW.vi"("invert"=w216, "step"=w227, "direction"=w228) -> ("CCW"=w217:bool, "CW"=w218:bool)  [unwired: 7 in]
      }
      frame True {
        n125 = case shown="True" w257 {
          tunnel: w256 -> [w267 w282]
          tunnel: [w267 w281] -> w255
          tunnel: w254 -> [w265 w280]
          tunnel: [w265 w279] -> w253
          tunnel: w252 -> [w263 w278]
          tunnel: [w263 w277] -> w251
          tunnel: w250 -> [w261 w276]
          tunnel: [w261 w275] -> w249
          tunnel: w248 -> [w259 w274]
          tunnel: [w259 w273] -> w247
          tunnel: w246 -> [w266 w272]
          tunnel: [w266 w272] -> w245
          tunnel: w244 -> [w264 w271]
          tunnel: [w264 w271] -> w243
          tunnel: w242 -> [w262 w270]
          tunnel: [w262 w270] -> w241
          tunnel: w240 -> [w260 w269]
          tunnel: [w260 w269] -> w239
          tunnel: w238 -> [w258 w268]
          tunnel: [w258 w268] -> w237
          frame False {
          }
          frame True {
            n126 = Not(x=w282) -> (.not. x?=w281:bool)
            n127 = Not(x=w280) -> (.not. x?=w279:bool)
            n128 = Not(x=w278) -> (.not. x?=w277:bool)
            n129 = Not(x=w276) -> (.not. x?=w275:bool)
            n130 = Not(x=w274) -> (.not. x?=w273:bool)
          }
        }
      }
    }
    n131 = xnode "FPGA I/O Node"("Axis1_CW"=w191, "Axis1_CCW"=w182, "Axis2_CW"=w190, "Axis2_CCW"=w189, "Axis3_CW"=w188, "Axis3_CCW"=w187, "Axis4_CW"=w186, "Axis4_CCW"=w185, "Axis5_CW"=w184, "Axis5_CCW"=w183) -> ()  [unwired: 10 in, 10 out]
  }
  n132 = timed-loop "Synchronization Loop" {
    timing: w6 -> [_]
    timing-out: [_] -> w5
    stop <- FALSE stop-if-true
    n133 = xnode "FPGA I/O Node"() -> ("Scan Clock"=w289:bool)  [unwired: 1 in, 1 out]
    n134 = global read "Global FPGA.vi" "Sync Enable"() -> (w288:bool)
    n135 = Select(t="Sync Value", s="Sync Enable override?", f=w288) -> (s? t:f=w285:bool)
    n136 = call-poly <vilib>:"nism.scan.generateSyncScan.vi"("Scan Enable?"=w285, "Scan Clock"=w289) -> ("Timer Control"=w290:T5)  [unwired: 3 in]
    n137 = global write "Global FPGA.vi" "Timer Control"(w290) -> ()
  }
  n138 = while {
    shift-right: [w296] -> _
    shift-left: FALSE ("RT Reset on Watchdog Failure?") -> [w295]
    stop <- FALSE stop-if-true
    # "Blink Loop"
    n139 = xnode "FPGA I/O Node"("FPGA LED"=w295) -> ()  [unwired: 1 in, 1 out]
    n140 = call "Wait"("Count(mSec)"=u8 100) -> ()  [unwired: 1 out]
    n141 = Not(x=w295) -> (.not. x?=w296:bool)
  }
  n142 = while "DIO Port A" {
    stop <- FALSE stop-if-true
    # "This implementation ended up not working...\nhad to pull out the digital filter."
    # "\"Reset I/O\""
    n143 = shared-variable "NI-sbRIO9606-018BB5CF\\User-Defined Variables\\Axis 1.DIO Control (Port A)"() -> (w313:u32)  [unwired: 1 in, 1 out]
    n144 = shared-variable "NI-sbRIO9606-018BB5CF\\User-Defined Variables\\Axis 2.DIO Control (Port A)"() -> (w312:u32)  [unwired: 1 in, 1 out]
    n145 = shared-variable "NI-sbRIO9606-018BB5CF\\User-Defined Variables\\Axis 3.DIO Control (Port A)"() -> (w311:u32)  [unwired: 1 in, 1 out]
    n146 = shared-variable "NI-sbRIO9606-018BB5CF\\User-Defined Variables\\Axis 4.DIO Control (Port A)"() -> (w310:u32)  [unwired: 1 in, 1 out]
    n147 = shared-variable "NI-sbRIO9606-018BB5CF\\User-Defined Variables\\Axis 5.DIO Control (Port A)"() -> (w309:u32)  [unwired: 1 in, 1 out]
    n148 = global read "Global FPGA.vi" "DIO Port A Config"() -> (w299:T10)
    n149 = Build Array(w313, w312, w311, w310, w309) -> (w308:u32[])
    n150 = for {
      tunnel: [w332] -> w307 mode=indexing
      tunnel: w308 -> [w331] mode=indexing
      tunnel: w299 -> [w321]
      tunnel: FALSE ("Reset I/O") -> [w319]
      tunnel: T9 {"reverse limit"=FALSE, "forward limit"=FALSE, "home switch"=FALSE, "digital input 0"=FALSE, "digital input 1"=FALSE, "digital input 2"=FALSE, "digital input 3"=FALSE} ("$(driveInterface.digitalInputs.shortName)") -> [w318]
      tunnel: "Axis Digital Inputs (U8)" -> [w315] mode=indexing
      # "#note Not reading the digital outputs for now,\njust using it for the \"latch\" number"
      n151 = Unbundle By Name(w321) -> ("digital filter (us)"=w329:u16[], "safe state"=w320:enum16{"Low", "High", "No Change"}[])
      n152 = call-poly <vilib>:"nism.digitalFilter.vi"("filter value (us)"=w329, "input signal"=w315) -> ("output signal"=w317:u8)  [unwired: 9 in]
      n153 = call-poly <vilib>:"nism.interpretDIOControl.portA.2.vi"("reset"=w319, "dio control(port a)"=w331, "safe state"=w320) -> ("reset latches"=w333:u8)  [unwired: 5 in, 1 out]
      n154 = Number To Boolean Array(number=w317) -> (Boolean array=w316:bool[])
      n155 = Index Array(array=w316) -> (element #1=w328:bool, element #2=w327:bool, element #3=w326:bool, element #4=w325:bool, element #5=w324:bool, element #6=w323:bool, element #7=w322:bool)  [unwired: 7 in]
      n156 = Bundle By Name(cluster=w318, "reverse limit"=w328, "forward limit"=w327, "home switch"=w326, "digital input 0"=w325, "digital input 1"=w324, "digital input 2"=w323, "digital input 3"=w322) -> (w330:T9)
      n157 = call-poly <vilib>:"nism.generateDIOStatus.portA.vi"("digital inputs"=w330, "reset latches"=w333) -> ("dio status(port a)"=w332:u32)  [unwired: 7 in]
    }
    n158 = Index Array(array=w307) -> (element #1=w306:u32, element #2=w305:u32, element #3=w304:u32, element #4=w303:u32, element #5=w302:u32)  [unwired: 5 in]
    n159 = shared-variable "NI-sbRIO9606-018BB5CF\\User-Defined Variables\\Axis 1.DIO Status (Port A)"(w306) -> ()  [unwired: 1 in, 1 out]
    n160 = shared-variable "NI-sbRIO9606-018BB5CF\\User-Defined Variables\\Axis 2.DIO Status (Port A)"(w305) -> ()  [unwired: 1 in, 1 out]
    n161 = shared-variable "NI-sbRIO9606-018BB5CF\\User-Defined Variables\\Axis 3.DIO Status (Port A)"(w304) -> ()  [unwired: 1 in, 1 out]
    n162 = shared-variable "NI-sbRIO9606-018BB5CF\\User-Defined Variables\\Axis 4.DIO Status (Port A)"(w303) -> ()  [unwired: 1 in, 1 out]
    n163 = shared-variable "NI-sbRIO9606-018BB5CF\\User-Defined Variables\\Axis 5.DIO Status (Port A)"(w302) -> ()  [unwired: 1 in, 1 out]
  }
  n164 = timed-loop "Reset Monitoring Loop" {
    timing: w4 -> [_]
    timing-out: [_] -> w3
    stop <- FALSE stop-if-true
    n165 = global read "Global FPGA.vi" "Reset Pending"() -> (w336:bool[])
    n166 = xnode "FPGA I/O Node"() -> ("Scan Clock"=w335:bool)  [unwired: 1 in, 1 out]
    n167 = feedback-in #1(w335) -> ()
    n168 = feedback #1() -> (w334:bool)  [unwired: 1 in]
    n169 = Greater?(x=w335, y=w334) -> (0:w340:bool)
    n170 = feedback #2() -> (w339:bool[])  [unwired: 1 in]
    n171 = Select(t=w336, s=w340, f=w339) -> (s? t:f=w337:bool[])
    n172 = feedback-in #2(w337) -> ()
    n173 = global write "Global FPGA.vi" "Reset"(w337) -> ()
  }
  n174 = node-c288(w3) -> ()
  n175 = node-c288(w5) -> ()
  n176 = node-c288(w7) -> ()
